vi "DAQmx Create Channel (AI-Temperature-RTD).vi"(0 "task in":refnum<k21>, 1 "maximum value":dbl=100.0 format="%0.2f", 2 "minimum value":dbl format="%0.2f", 3 "resistance configuration":i32(ring)=2 items=["2-Wire"=2, "3-Wire"=3, "4-Wire"=4], 5 "physical channels":tag, 6 "r0":dbl=100.0 format="%0.2f", 7 "name to assign":string, 9 "units":i32(ring)=10143 items=["Deg C"=10143, "Deg F"=10144, "Kelvins"=10325, "Deg R"=10145, "From Custom Scale"=10065], 10 "current excitation value":dbl=0.0025 format="%0.5f", 11 "error in":errorcluster, 13 "current excitation source":i32(ring)=10167 items=["Internal"=10200, "External"=10167, "None"=10230], 14 "rtd type":i32(ring)=12481 items=["Pt3750"=12481, "Pt3851"=10071, "Pt3911"=12482, "Pt3916"=10069, "Pt3920"=10053, "Pt3928"=12483, "Custom"=10137]) -> (4 "task out":refnum<k21>, 15 "error out":errorcluster)   [LabVIEW 2020]
doc: "Creates channel(s) that use an RTD to measure temperature."
uses:
  nilvaiu.dll
panel:
  # "input limits"
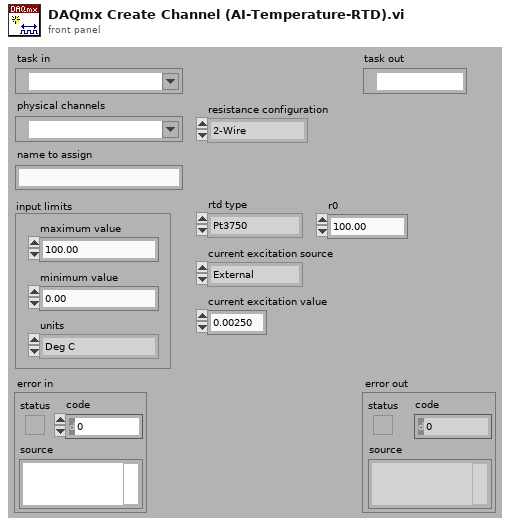
[diagram p1: front panel]
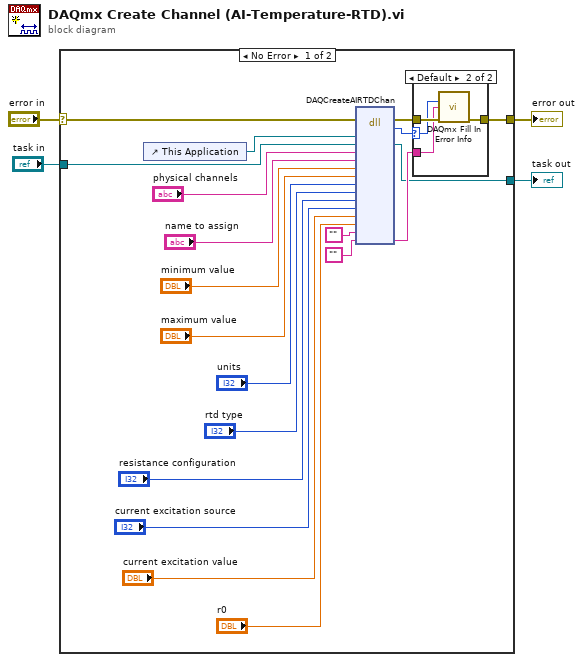
[diagram p0: block diagram]
diagram:
  n1 = case shown="No Error" "error in" {
    selector: "error in" -> [w8 w31]
    tunnel: "task in" -> [w10 w30]
    tunnel: [w9 w30] -> w3
    tunnel: [w7 w31] -> w1
    frame No Error {
      n2 = control-ref of="This Application"() -> (w11:refnum<vi>)
      n3 = dll-call lib="nilvaiu.*" fn="DAQCreateAIRTDChan"(error in=w8, "lvAppRef"=w11, "refObjPtr"=w10, "physicalChannelName"="physical channels", "channelNameIn"="name to assign", "minVal"="minimum value", "maxVal"="maximum value", "units"="units", "rtdType"="rtd type", "resistanceConfiguration"="resistance configuration", "currentExcitSource"="current excitation source", "currentExcitVal"="current excitation value", "r0"="r0", "channelNamesOut"="", "extendedErrorInfo"="") -> (error out=w24:errorcluster, "return type"=w23:i32, "refObjPtr"=w9:refnum<k21>, "extendedErrorInfo"=w22:string)  [unwired: 14 in, 1 out]
      n4 = case shown="Default" w23 {
        selector: w23 -> [_ w27]
        tunnel: w24 -> [w25 w29]
        tunnel: [w25 w28] -> w7
        tunnel: w22 -> [_ w26]
        frame 0 {
        }
        frame Default {
          n5 = call "DAQmx Fill In Error Info.vi"("status code"=w27, "extended error info"=w26, "error in"=w29) -> ("error out"=w28:errorcluster)  [unwired: 1 in, 11 out]
        }
      }
    }
    frame Error {
    }
  }
  "task out" <- w3
  "error out" <- w1
